vi "GetFPGA1212Reference.vi"(2 "error in":errorcluster, 3 "RIO Device IN":T1="RIO0" caption="RIO Device") -> (0 "error out":errorcluster, 1 "FPGA VI Reference Out":refnum<k20>)   [LabVIEW 2018]
uses:
  <vilib>/userdefined/High Color/nirio_resource_hc.ctl
  <vilib>/rvi/interface/RandomDataEmulation/nirviRandomDataOpen.vi
  <vilib>/rvi/interface/common/niFpgaCacheSessionInfoDynamic.vi
  GlobalAT_SigGen.vi
  <vilib>/rvi/interface/nirviOpenFPGA/nirviOpenFPGA.xnode
  D:/HardwareRevamp/AcustoXv2/FPGA/Generator1212/ReadWriteTablesTest_1212_K7.vi
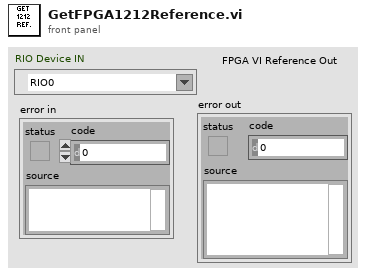
[diagram p1: front panel]
types:
  T1 = typedef "nirio_resource_hc.ctl" = tag
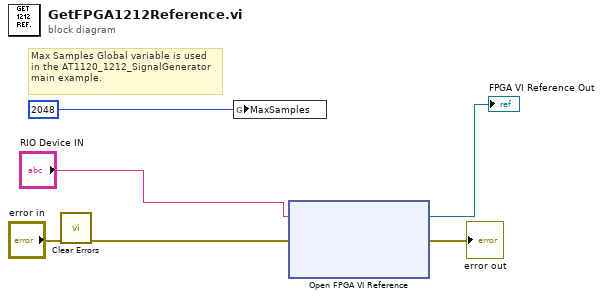
[diagram p0: block diagram]
diagram:
  # "Max Samples Global variable is used\nin the AT1120_1212_SignalGenerator\nmain example."
  n1 = call <vilib>:"Clear Errors.vi"("error in (no error)"="error in") -> ("error out"=w1:errorcluster)  [unwired: 5 in, 1 out]
  n2 = global write "GlobalAT_SigGen.vi" "MaxSamples"(u16 2048 ("MaxSamples")) -> ()
  n3 = xnode "Open FPGA VI Reference"("error in"=w1, "resource name"="RIO Device IN") -> ("FPGA VI Reference Out"=→"FPGA VI Reference Out":refnum<k20>, "error out"=→"error out":errorcluster)
